vi "Do.vi"(8 "error in (no error)":errorcluster, 10 "Actor in":refnum<class "Actor.lvclass">, 11 "Launch Nested Models Msg":refnum<class "Auto-Launch Models Msg.lvclass">) -> (0 "error out":errorcluster, 2 "Actor out":refnum<class "Actor.lvclass">)   [LabVIEW 2017, in "IModel.lvlib" / "Auto-Launch Models Msg.lvclass"]
doc: "This VI delivers the message to the actor by calling the appropriate method(s) on the actor."
uses:
  <vilib>/gpm_packages/@cs/mva-core/Source/IModel/IModel Messages/Auto-Launch Models Msg/Auto-Launch Models Msg.lvclass
  <vilib>/ActorFramework/Actor/Actor.lvclass
  <vilib>/gpm_packages/@cs/mva-core/Source/IModel/IModel/IModel.lvclass
  C:/Program Files/National Instruments/LabVIEW 2017/vi.lib/ActorFramework/Actor/Actor.lvclass
  <vilib>/gpm_packages/@cs/mva-core/Source/IModel/IModel Messages/Auto-Launch Models Msg/Auto-Launch Models Msg.lvclass/Auto-Launch Models Msg.ctl
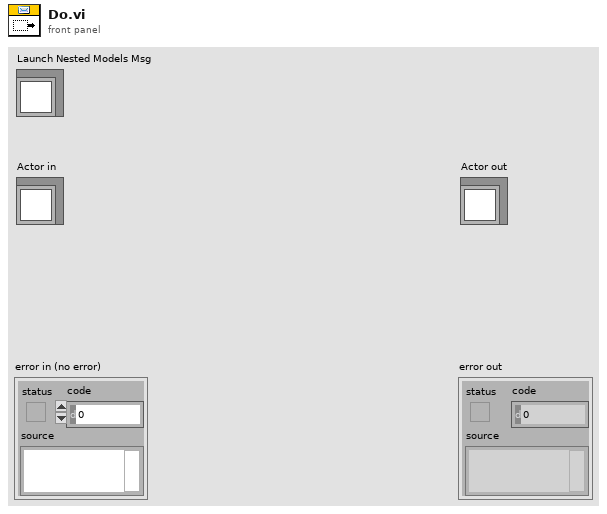
[diagram p1: front panel]
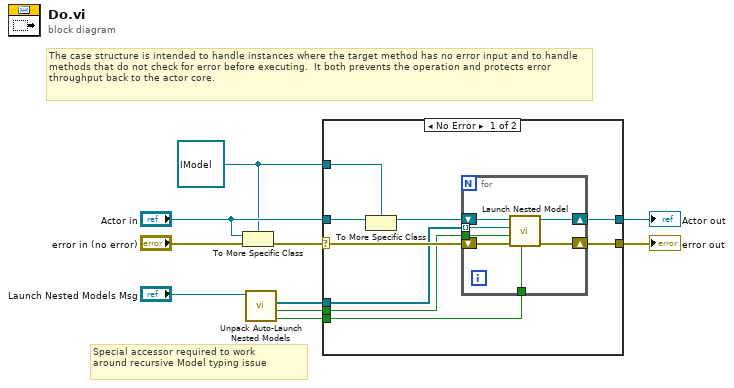
[diagram p0: block diagram]
diagram:
  w5 = refnum<class "IModel.lvclass"> refnum ("Actor in")
  # "Special accessor required to work\naround recursive Model typing issue"
  # "The case structure is intended to handle instances where the target method has no error input and to handle methods that do not check for error before executing.  It both prevents the operation and protects error throughput back to the actor core."
  n1 = To More Specific Class(target class=w5, reference="Actor in", error in="error in (no error)") -> (error out=w9:errorcluster)  [unwired: 1 out]
  n2 = call <vilib>:"Unpack Auto-Launch Nested Models.vi"("Launch Nested Models Msg"="Launch Nested Models Msg") -> ("Confirm Shutdown? (T)"=w1:bool, "Auto-stop? (T)"=w2:bool, "Nested Models"=w3:refnum<class "IModel.lvclass">[])  [unwired: 8 in]
  n3 = case shown="No Error" w9 {
    selector: w9 -> [w17 w28]
    tunnel: [w19 w28] -> w8
    tunnel: [w18 w27] -> w7
    tunnel: "Actor in" -> [w16 w27]
    tunnel: w5 -> [w15 _]
    tunnel: w3 -> [w13 _]
    tunnel: w2 -> [w12 _]
    tunnel: w1 -> [w11 _]
    frame No Error {
      n4 = To More Specific Class(target class=w15, reference=w16) -> (specific class reference=w14:refnum<class "IModel.lvclass">)  [unwired: 1 in, 1 out]
      n5 = for {
        tunnel: w13 -> [w22] mode=indexing
        shift-right: [w26] -> w19
        shift-left: w17 -> [w24]
        shift-right: [w25] -> w18
        shift-left: w14 -> [w23]
        tunnel: w12 -> [w21]
        tunnel: w11 -> [w20]
        n6 = call-dynamic "Launch Nested Model.vi"("Confirm Shutdown? (T)"=w20, "error in (no error)"=w24, "Auto-stop? (T)"=w21, "Model to Launch"=w22, "IModel in"=w23) -> ("error out"=w26:errorcluster, "IModel out"=w25:refnum<class "IModel.lvclass">)  [unwired: 4 in, 1 out]
      }
    }
    frame Error {
      # "If type check fails, pass the\noriginal object out again."
    }
  }
  "error out" <- w8
  "Actor out" <- w7
